vi "Motor and Sensor.vi"() -> ()   [LabVIEW 2019]
uses:
  <vilib>/Instr/_visa.llb/VISA Configure Serial Port (Instr).vi
panel:
  in  "Zero1":dbl
  in  "Zero2":dbl
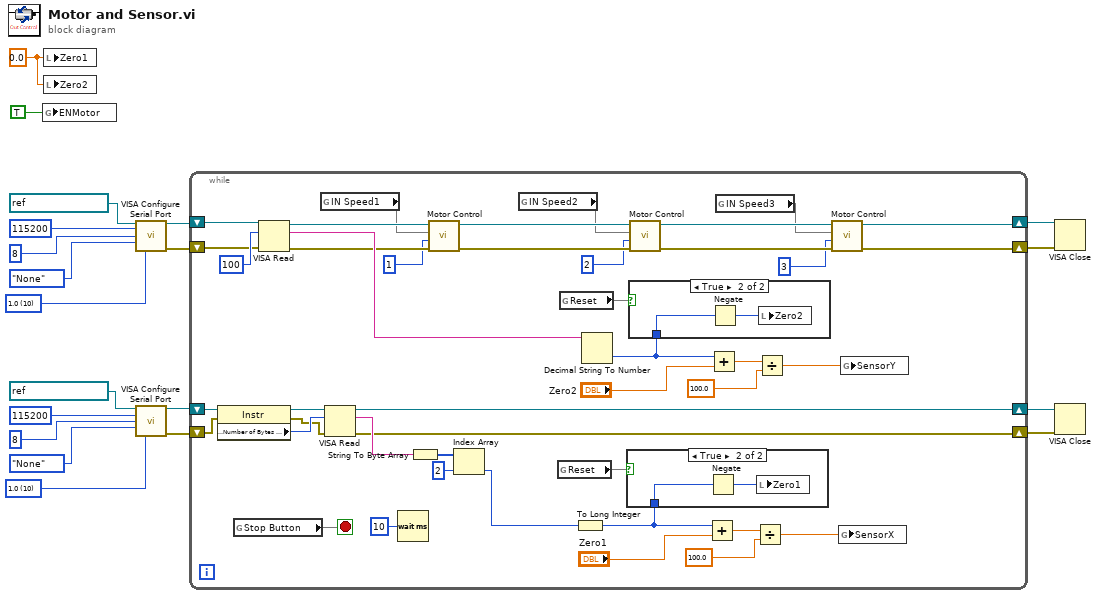
[diagram p0: block diagram]
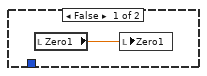
[diagram p2: hidden frame]
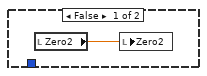
[diagram p3: hidden frame]
diagram:
  w1 = 0.0 ("Zero1")
  w13 = u16 10 items=["1.0"=10, "1.5"=15, "2.0"=20] ("stop bits (10: 1 bit)")
  w18 = u16 10 items=["1.0"=10, "1.5"=15, "2.0"=20] ("stop bits (10: 1 bit)")
  n1 = global write "Motor Control.vi" "ENMotor"(TRUE ("ENMotor")) -> ()
  n2 = local write "Zero1"(w1) -> ()
  n3 = local write "Zero2"(w1) -> ()
  n4 = call-poly "VISA Configure Serial Port"("VISA resource name"=refnum<visa-resource-name> "ASRL1::INSTR", "baud rate (9600)"=u32 115200, "data bits (8)"=u16 8, "parity (0:none)"=enum16{"None", "Odd", "Even", "Mark", "Space"}."None", "stop bits (10: 1 bit)"=w18) -> ("VISA resource name out"=w10:refnum<visa-resource-name>, "error out"=w9:errorcluster)  [unwired: 9 in]
  n5 = call-poly "VISA Configure Serial Port"("VISA resource name"=refnum<visa-resource-name> "ASRL2::INSTR", "baud rate (9600)"=u32 115200, "data bits (8)"=u16 8, "parity (0:none)"=enum16{"None", "Odd", "Even", "Mark", "Space"}."None", "stop bits (10: 1 bit)"=w13) -> ("VISA resource name out"=w8:refnum<visa-resource-name>, "error out"=w7:errorcluster)  [unwired: 9 in]
  n6 = while {
    shift-right: [w24] -> w3
    shift-left: w10 -> [w26]
    shift-right: [w23] -> w4
    shift-left: w9 -> [w25]
    shift-right: [w22] -> w5
    shift-left: w8 -> [w27]
    shift-right: [w21] -> w6
    shift-left: w7 -> [w28]
    stop <- w62 stop-if-true
    n7 = property class="Instr"(reference=w27, error in=w28) -> (reference out=w46:refnum<visa-resource-name>, error out=w43:errorcluster, "Serial Settings:Number of Bytes at Serial Port"=w45:u32)
    n8 = global read "Motor Control.vi" "Stop Button"() -> (w62)
    n9 = VISA Read(VISA resource name=w26, byte count=u32 100, error in (no error)=w25) -> (VISA resource name out=w55:refnum<visa-resource-name>, read buffer=w59:string, error out=w56:errorcluster)  [unwired: 1 out]
    n10 = global read "Motor Control.vi" "IN Speed1"() -> (w50)
    n11 = VISA Read(VISA resource name=w46, byte count=w45, error in (no error)=w43) -> (VISA resource name out=w22:refnum<visa-resource-name>, read buffer=w47:string, error out=w21:errorcluster)  [unwired: 1 out]
    n12 = Wait (ms)(milliseconds to wait=u32 10) -> ()  [unwired: 1 out]
    n13 = String To Byte Array(string=w47) -> (unsigned byte array=w44:u8[])
    n14 = call "Motor Control.vi"("error in (no error)"=w56, "MotorSelect"=i16 1, "INSpeed"=w50, "VISA Refnum in"=w55) -> ("error out"=w53:errorcluster, "VISA Refnum out"=w54:refnum<visa-resource-name>)  [unwired: 6 in]
    n15 = Index Array(array=w44, index=2) -> (element=w38:u8)
    n16 = global read "Motor Control.vi" "IN Speed2"() -> (w49)
    n17 = global read "Motor Control.vi" "Reset"() -> (w42)
    n18 = global read "Motor Control.vi" "Reset"() -> (w61)
    n19 = To Long Integer(number=w38) -> (32bit integer=w39:i32)
    n20 = Decimal String To Number(string=w59) -> (number=w60:i32)  [unwired: 2 in, 1 out]
    n21 = case shown="True" w42 {
      tunnel: w39 -> [_ w65]
      frame False {
        n22 = local read "Zero1"() -> (w64:dbl)
        n23 = local write "Zero1"(w64) -> ()
      }
      frame True {
        n24 = Negate(x=w65) -> (-x=w66:i32)
        n25 = local write "Zero1"(w66) -> ()
      }
    }
    n26 = case shown="True" w61 {
      tunnel: w60 -> [_ w68]
      frame False {
        n27 = local read "Zero2"() -> (w67:dbl)
        n28 = local write "Zero2"(w67) -> ()
      }
      frame True {
        n29 = Negate(x=w68) -> (-x=w69:i32)
        n30 = local write "Zero2"(w69) -> ()
      }
    }
    n31 = call "Motor Control.vi"("error in (no error)"=w53, "MotorSelect"=i16 2, "INSpeed"=w49, "VISA Refnum in"=w54) -> ("error out"=w51:errorcluster, "VISA Refnum out"=w52:refnum<visa-resource-name>)  [unwired: 6 in]
    n32 = Add(x=w39, y="Zero1") -> (x+y=w40:dbl)
    n33 = Add(x=w60, y="Zero2") -> (x+y=w57:dbl)
    n34 = global read "Motor Control.vi" "IN Speed3"() -> (w48)
    n35 = Divide(x=w40, y=100.0) -> (x/y=w37:dbl)
    n36 = Divide(x=w57, y=100.0) -> (x/y=w36:dbl)
    n37 = call "Motor Control.vi"("error in (no error)"=w51, "MotorSelect"=i16 3, "INSpeed"=w48, "VISA Refnum in"=w52) -> ("error out"=w23:errorcluster, "VISA Refnum out"=w24:refnum<visa-resource-name>)  [unwired: 6 in]
    n38 = global write "Motor Control.vi" "SensorX"(w37) -> ()
    n39 = global write "Motor Control.vi" "SensorY"(w36) -> ()
  }
  n40 = VISA Close(VISA resource name=w3, error in (no error)=w4) -> ()  [unwired: 1 out]
  n41 = VISA Close(VISA resource name=w5, error in (no error)=w6) -> ()  [unwired: 1 out]
